vi "getCamReference.vi"(8 "error in (no error)":errorcluster, 11 "ICCameraController in":refnum<class "ICCameraController.lvclass">) -> (0 "error out":errorcluster, 2 "ICImagingControlRef":refnum<k7>, 3 "ICCameraController out":refnum<class "ICCameraController.lvclass">)   [LabVIEW 2011, in "Hardware.lvlib" / "Channels.lvlib" / "ICCameraController.lvclass"]
uses:
  ICCameraController.lvclass
  ICCameraController.lvclass/ICCameraController.ctl
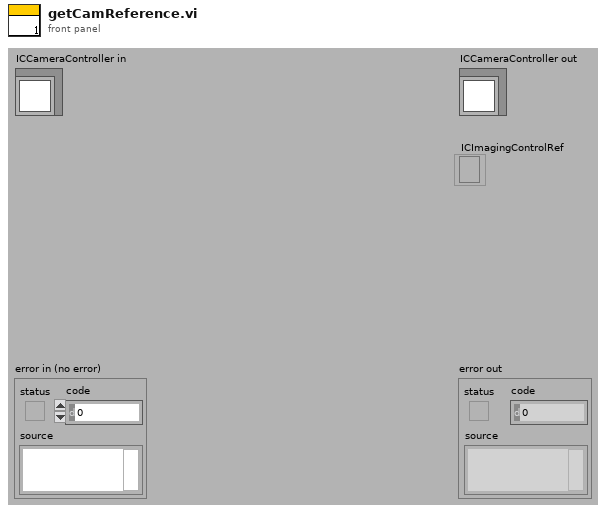
[diagram p1: front panel]
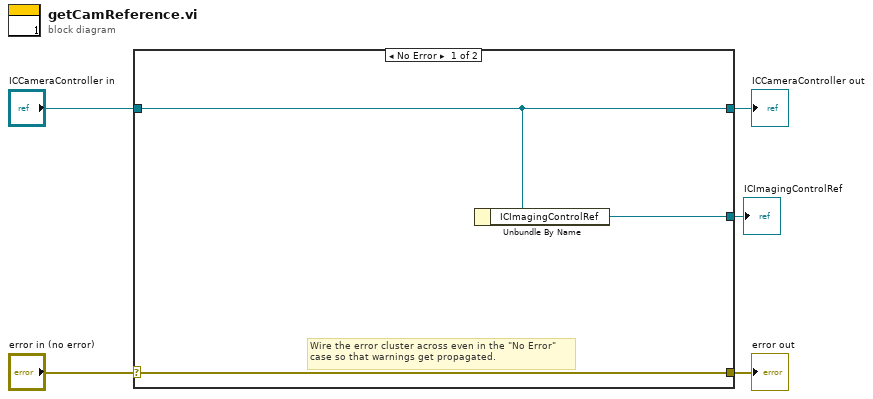
[diagram p0: block diagram]
diagram:
  n1 = case shown="No Error" "error in (no error)" {
    selector: "error in (no error)" -> [w8 w10]
    tunnel: [w8 w10] -> w4
    tunnel: [w7 w9] -> w2
    tunnel: "ICCameraController in" -> [w7 w9]
    tunnel: [w6 _] -> w1
    frame No Error {
      # "Wire the error cluster across even in the \"No Error\"\ncase so that warnings get propagated."
      n2 = Unbundle By Name(w7) -> ("ICImagingControlRef"=w6:refnum<k7>)
    }
    frame Error {
    }
  }
  "error out" <- w4
  "ICCameraController out" <- w2
  "ICImagingControlRef" <- w1
